vi "Client_Create.vi"(0 "reference in":refnum<class "Client.lvclass">, 5 "Device ID":u32, 11 "Error In":errorcluster) -> (4 "reference out":refnum<class "Client.lvclass">, 15 "Error Out":errorcluster)   [LabVIEW 2024, in "Client.lvclass"]
uses:
  Client.lvclass
  Receiver/MediaPlayer_class/MediaPlayer.lvclass
  Invoker/RemoteControl_class/RemoteControl.lvclass
  Commands/PlayMusicCommand_class/PlayMusicCommand.lvclass
  Commands/PauseMusicCommand_class/PauseMusicCommand.lvclass
  Commands/StopMusicCommand_class/StopMusicCommand.lvclass
  Commands/SkipMusicCommand_class/SkipMusicCommand.lvclass
  Commands/GetCurrentInfoCommand_class/GetCurrentInfoCommand.lvclass
  Commands/RewindMusicCommand_class/RewindMusicCommand.lvclass
  Client.lvclass/Client.ctl
panel:
  # "Connector Pane"
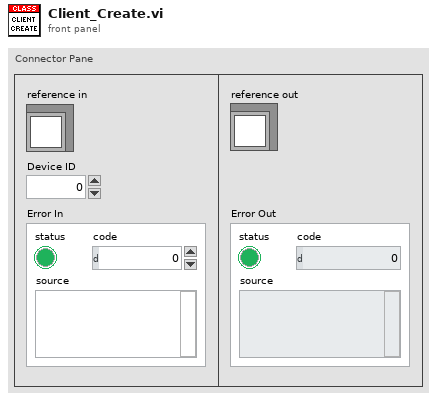
[diagram p1: front panel]
types:
  T1 = typedef "Client.lvclass/ObjectAttributes.ctl" = cluster{"RemoteControlRef":refnum<class "RemoteControl.lvclass">, "MediaPlayerRef":refnum<class "MediaPlayer.lvclass">, "Commands":cluster{"Play Music Command":refnum<class "IPlayerCommand.lvclass">, "Pause Music Command":refnum<class "IPlayerCommand.lvclass">, "Stop Music Command":refnum<class "IPlayerCommand.lvclass">, "Skip Music Command":refnum<class "IPlayerCommand.lvclass">, "Get Current Info Command":refnum<class "IPlayerCommand.lvclass">, "Rewind Music Command":refnum<class "IPlayerCommand.lvclass">}}
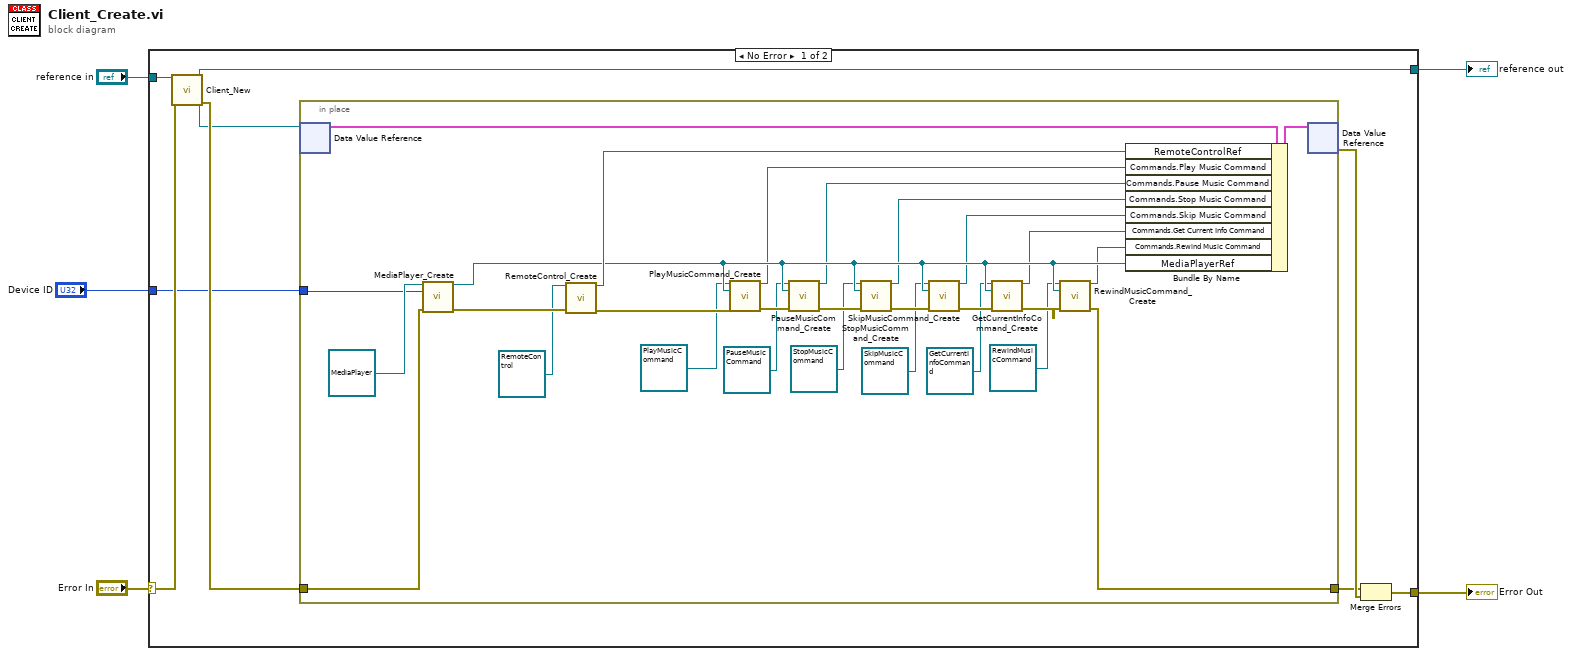
[diagram p0: block diagram]
diagram:
  n1 = case shown="No Error" "Error In" {
    selector: "Error In" -> [w8 w44]
    tunnel: [w10 w44] -> w4
    tunnel: "reference in" -> [w9 w43]
    tunnel: [w14 w43] -> w2
    tunnel: "Device ID" -> [w6 _]
    frame No Error {
      n2 = call "Client_New.vi"("reference in"=w9, "Error In"=w8) -> ("reference out"=w14:refnum<class "Client.lvclass">, "DVRRefOut"=w7:refnum<data-value>, "Error Out"=w12:errorcluster)  [unwired: 10 in, 1 out]
      n3 = in-place {
        in-place-border: w12 -> [w36]
        in-place-border: [w16] -> w11
        in-place-border: w6 -> [w15]
        n4 = in-place-dvr #1(w7) -> (w41:T1)  [unwired: 1 out]
        n5 = call "MediaPlayer_Create.vi"("reference in"=refnum<class "MediaPlayer.lvclass"> refnum ("MediaPlayer"), "Device ID"=w15, "Error In"=w36) -> ("reference out"=w34:refnum<class "MediaPlayer.lvclass">, "Error Out"=w40:errorcluster)  [unwired: 11 in]
        n6 = call "RemoteControl_Create.vi"("reference in"=refnum<class "RemoteControl.lvclass"> refnum ("RemoteControl"), "Error In"=w40) -> ("reference out"=w37:refnum<class "RemoteControl.lvclass">, "Error Out"=w35:errorcluster)  [unwired: 12 in]
        n7 = call "PlayMusicCommand_Create.vi"("reference in"=refnum<class "PlayMusicCommand.lvclass"> refnum ("PlayMusicCommand"), "MediaPlayer"=w34, "Error In"=w35) -> ("reference out"=w26:refnum<class "PlayMusicCommand.lvclass">, "Error Out"=w33:errorcluster)  [unwired: 11 in]
        n8 = call "PauseMusicCommand_Create.vi"("reference in"=refnum<class "PauseMusicCommand.lvclass"> refnum ("PauseMusicCommand"), "MediaPlayer"=w34, "Error In"=w33) -> ("reference out"=w25:refnum<class "PauseMusicCommand.lvclass">, "Error Out"=w32:errorcluster)  [unwired: 11 in]
        n9 = call "StopMusicCommand_Create.vi"("reference in"=refnum<class "StopMusicCommand.lvclass"> refnum ("StopMusicCommand"), "MediaPlayer"=w34, "Error In"=w32) -> ("reference out"=w20:refnum<class "StopMusicCommand.lvclass">, "Error Out"=w31:errorcluster)  [unwired: 11 in]
        n10 = call "SkipMusicCommand_Create.vi"("reference in"=refnum<class "SkipMusicCommand.lvclass"> refnum ("SkipMusicCommand"), "MediaPlayerRef"=w34, "Error In"=w31) -> ("reference out"=w19:refnum<class "SkipMusicCommand.lvclass">, "Error Out"=w30:errorcluster)  [unwired: 11 in]
        n11 = call "GetCurrentInfoCommand_Create.vi"("reference in"=refnum<class "GetCurrentInfoCommand.lvclass"> refnum ("GetCurrentInfoCommand"), "MediaPlayerRef"=w34, "Error In"=w30) -> ("reference out"=w18:refnum<class "GetCurrentInfoCommand.lvclass">, "Error Out"=w29:errorcluster)  [unwired: 11 in]
        n12 = call "RewindMusicCommand_Create.vi"("reference in"=refnum<class "RewindMusicCommand.lvclass"> refnum ("RewindMusicCommand"), "MediaPlayerRef"=w34, "Error In"=w29) -> ("reference out"=w17:refnum<class "RewindMusicCommand.lvclass">, "Error Out"=w16:errorcluster)  [unwired: 11 in]
        n13 = Bundle By Name(cluster=w41, "RemoteControlRef"=w37, "Commands.Play Music Command"=w26, "Commands.Pause Music Command"=w25, "Commands.Stop Music Command"=w20, "Commands.Skip Music Command"=w19, "Commands.Get Current Info Command"=w18, "Commands.Rewind Music Command"=w17, "MediaPlayerRef"=w34) -> (w42:T1)
        n14 = in-place-dvr #1(w42) -> (w13:errorcluster)  [unwired: 1 out]
      }
      n15 = Merge Errors(w11, w13) -> (w10:errorcluster)
    }
    frame Error {
      # "VI-TechBaseTemplate_Simple_4x4x4"
    }
  }
  "Error Out" <- w4
  "reference out" <- w2
